vi "Graph Utilities Tree.vi"() -> ()   [LabVIEW 2016, in "graph_utilities.lvclass"]
uses:
  graph_utilities.lvclass
  graph_utilities.lvclass/graph_utilities.ctl
panel:
  out "XY Graph":cluster{"Intensity Data":dbl[], "Array":dbl[]}[](graph)
  out "Intensity Graph":dbl[][](graph)
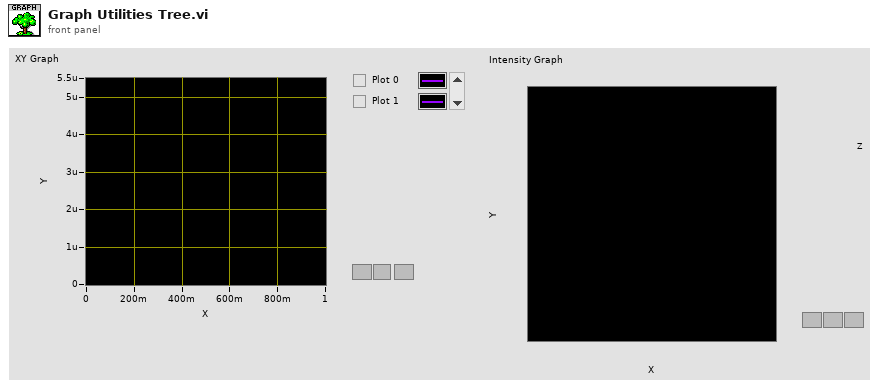
[diagram p1: front panel]
types:
  T1 = typedef "LVPointDoubleTypeDef.ctl" = cluster{"X":dbl, "Y":dbl}
  T2 = typedef "graph_utilities.lvclass/Scale Mapping  - Enum.ctl" = u16
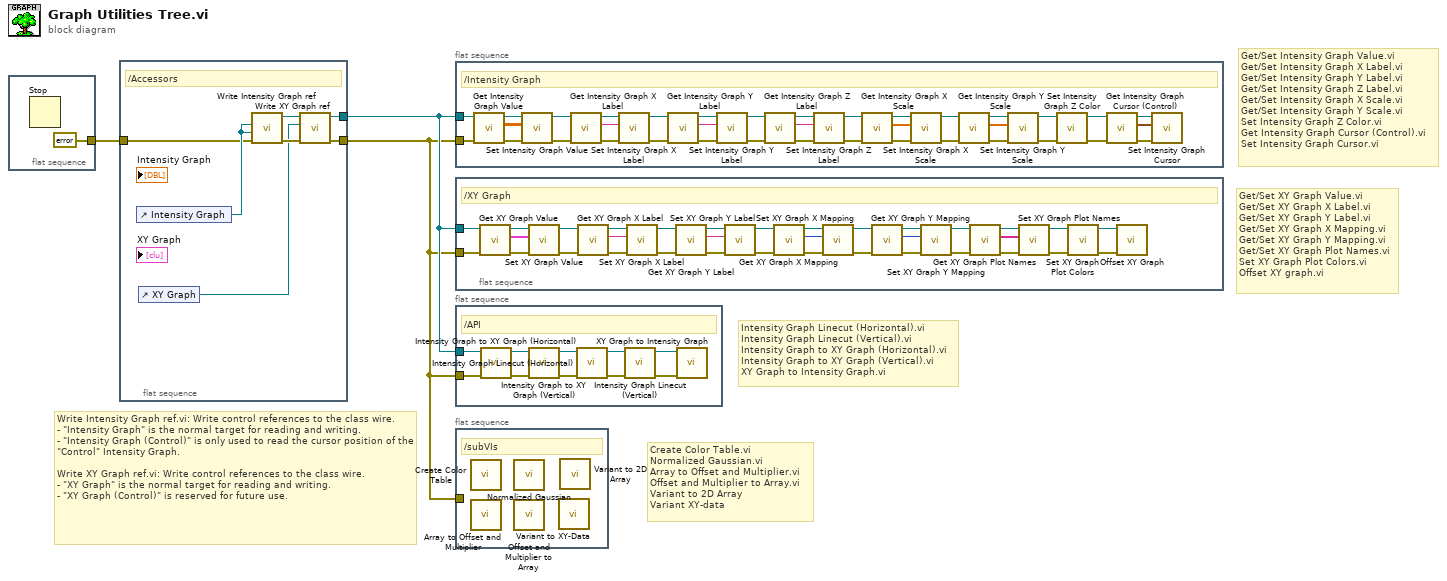
[diagram p0: block diagram]
diagram:
  # "Create Color Table.vi\nNormalized Gaussian.vi\nArray to Offset and Multiplier.vi\nOffset and Multiplier to Array.vi\nVariant to 2D Array\nVariant XY-data"
  # "Write Intensity Graph ref.vi: Write control references to the class wire.\n- \"Intensity Graph\" is the normal target for reading and writing.\n- \"Intensity Graph (Control)\" is only used to read the cursor position of the \"Control\" Intensity Graph.\n\nWrite XY Graph ref.vi: Write control references to the class wire.\n- \"XY Graph\" is the normal target for reading and writing.\n- \"XY Graph (Control)\" is reserved for future use."
  # "Get/Set Intensity Graph Value.vi\nGet/Set Intensity Graph X Label.vi\nGet/Set Intensity Graph Y Label.vi\nGet/Set Intensity Graph Z Label.vi\nGet/Set Intensity Graph X Scale.vi\nGet/Set Intensity Graph Y Scale.vi\nSet Intensity Graph Z Color.vi\nGet Intensity Graph Cursor (Control).vi\nSet Intensity Graph Cursor.vi"
  # "Get/Set XY Graph Value.vi\nGet/Set XY Graph X Label.vi\nGet/Set XY Graph Y Label.vi\nGet/Set XY Graph X Mapping.vi\nGet/Set XY Graph Y Mapping.vi\nGet/Set XY Graph Plot Names.vi\nSet XY Graph Plot Colors.vi\nOffset XY graph.vi"
  # "Intensity Graph Linecut (Horizontal).vi\nIntensity Graph Linecut (Vertical).vi\nIntensity Graph to XY Graph (Horizontal).vi\nIntensity Graph to XY Graph (Vertical).vi\nXY Graph to Intensity Graph.vi"
  n1 = flat-sequence {
    tunnel: [errorcluster {"status"=FALSE, "code"=0, "source"=""} ("error in (no error)")] -> w3
    frame #0 {
      n2 = Stop() -> ()  [unwired: 1 in]
    }
  }
  n3 = flat-sequence {
    tunnel: w3 -> [w7]
    tunnel: [w6] -> w2
    tunnel: [w5] -> w1
    frame #0 {
      # "/Accessors"
      n4 = control-ref of="Intensity Graph"() -> (w8:refnum<vi>)
      n5 = control-ref of="XY Graph"() -> (w9:refnum<vi>)
      n6 = call "Write Intensity Graph ref.vi"("error in (no error)"=w7, "Intensity Graph (Control)"=w8, "Intensity Graph"=w8) -> ("error out"=w10:errorcluster, "graph_utilities out"=w11:refnum<class "graph_utilities.lvclass">)  [unwired: 7 in]
      n7 = call "Write XY Graph ref.vi"("error in (no error)"=w10, "XY Graph"=w9, "graph_utilities in"=w11) -> ("error out"=w5:errorcluster, "graph_utilities out"=w6:refnum<class "graph_utilities.lvclass">)  [unwired: 7 in]
    }
  }
  n8 = flat-sequence {
    tunnel: w2 -> [w13]
    tunnel: w1 -> [w12]
    frame #0 {
      # "/Intensity Graph"
      n9 = call "Get Intensity Graph Value.vi"("error in (no error)"=w12, "graph_utilities in"=w13) -> ("error out"=w46:errorcluster, "Value"=w48:dbl[][], "graph_utilities out"=w47:refnum<class "graph_utilities.lvclass">)  [unwired: 7 in]
      n10 = call "Set Intensity Graph Value.vi"("error in (no error)"=w46, "Value"=w48, "graph_utilities in"=w47) -> ("error out"=w44:errorcluster, "graph_utilities out"=w45:refnum<class "graph_utilities.lvclass">)  [unwired: 7 in]
      n11 = call "Get Intensity Graph X Label.vi"("error in (no error)"=w44, "graph_utilities in"=w45) -> ("error out"=w42:errorcluster, "X Label"=w23:string, "graph_utilities out"=w43:refnum<class "graph_utilities.lvclass">)  [unwired: 7 in]
      n12 = call "Set Intensity Graph X Label.vi"("error in (no error)"=w42, "X Label"=w23, "graph_utilities in"=w43) -> ("error out"=w40:errorcluster, "graph_utilities out"=w41:refnum<class "graph_utilities.lvclass">)  [unwired: 7 in]
      n13 = call "Get Intensity Graph Y Label.vi"("error in (no error)"=w40, "graph_utilities in"=w41) -> ("error out"=w38:errorcluster, "Y Label"=w22:string, "graph_utilities out"=w39:refnum<class "graph_utilities.lvclass">)  [unwired: 7 in]
      n14 = call "Set Intensity Graph Y Label.vi"("error in (no error)"=w38, "Y Label"=w22, "graph_utilities in"=w39) -> ("error out"=w36:errorcluster, "graph_utilities out"=w37:refnum<class "graph_utilities.lvclass">)  [unwired: 7 in]
      n15 = call "Get Intensity Graph Z Label.vi"("error in (no error)"=w36, "graph_utilities in"=w37) -> ("error out"=w34:errorcluster, "Z Label"=w21:string, "graph_utilities out"=w35:refnum<class "graph_utilities.lvclass">)  [unwired: 7 in]
      n16 = call "Set Intensity Graph Z Label.vi"("error in (no error)"=w34, "Z Label"=w21, "graph_utilities in"=w35) -> ("error out"=w32:errorcluster, "graph_utilities out"=w33:refnum<class "graph_utilities.lvclass">)  [unwired: 7 in]
      n17 = call "Get Intensity Graph X Scale.vi"("error in (no error)"=w32, "graph_utilities in"=w33) -> ("error out"=w30:errorcluster, "X Scale"=w20:dbl[], "graph_utilities out"=w31:refnum<class "graph_utilities.lvclass">)  [unwired: 6 in, 1 out]
      n18 = call "Set Intensity Graph X Scale.vi"("error in (no error)"=w30, "X Scale"=w20, "graph_utilities in"=w31) -> ("error out"=w28:errorcluster, "graph_utilities out"=w29:refnum<class "graph_utilities.lvclass">)  [unwired: 7 in]
      n19 = call "Get Intensity Graph Y Scale.vi"("error in (no error)"=w28, "graph_utilities in"=w29) -> ("error out"=w26:errorcluster, "Y Scale"=w19:dbl[], "graph_utilities out"=w27:refnum<class "graph_utilities.lvclass">)  [unwired: 6 in, 1 out]
      n20 = call "Set Intensity Graph Y Scale.vi"("error in (no error)"=w26, "Y Scale"=w19, "graph_utilities in"=w27) -> ("error out"=w24:errorcluster, "graph_utilities out"=w25:refnum<class "graph_utilities.lvclass">)  [unwired: 7 in]
      n21 = call "Set Intensity Graph Z Color.vi"("error in (no error)"=w24, "graph_utilities in"=w25) -> ("error out"=w17:errorcluster, "graph_utilities out"=w16:refnum<class "graph_utilities.lvclass">)  [unwired: 8 in]
      n22 = call "Get Intensity Graph Cursor (Control).vi"("error in (no error)"=w17, "graph_utilities in"=w16) -> ("error out"=w15:errorcluster, "Cursor.Cursor Position"=w18:T1, "graph_utilities out"=w14:refnum<class "graph_utilities.lvclass">)  [unwired: 7 in]
      n23 = call "Set Intensity Graph Cursor.vi"("error in (no error)"=w15, "Cursor.Cursor Position"=w18, "graph_utilities in"=w14) -> ()  [unwired: 7 in, 2 out]
    }
  }
  n24 = flat-sequence {
    tunnel: w2 -> [w69]
    tunnel: w1 -> [w68]
    frame #0 {
      # "/XY Graph"
      n25 = call "Get XY Graph Value.vi"("error in (no error)"=w68, "graph_utilities in"=w69) -> ("error out"=w80:errorcluster, "Value"=w82:cluster{"X":dbl[], "Y":dbl[]}[], "graph_utilities out"=w81:refnum<class "graph_utilities.lvclass">)  [unwired: 7 in]
      n26 = call "Set XY Graph Value.vi"("error in (no error)"=w80, "Value"=w82, "graph_utilities in"=w81) -> ("error out"=w78:errorcluster, "graph_utilities out"=w79:refnum<class "graph_utilities.lvclass">)  [unwired: 7 in]
      n27 = call "Get XY Graph X Label.vi"("error in (no error)"=w78, "graph_utilities in"=w79) -> ("error out"=w76:errorcluster, "X Label"=w70:string, "graph_utilities out"=w77:refnum<class "graph_utilities.lvclass">)  [unwired: 7 in]
      n28 = call "Set XY Graph X Label.vi"("error in (no error)"=w76, "X Label"=w70, "graph_utilities in"=w77) -> ("error out"=w74:errorcluster, "graph_utilities out"=w75:refnum<class "graph_utilities.lvclass">)  [unwired: 7 in]
      n29 = call "Get XY Graph Y Label.vi"("error in (no error)"=w74, "graph_utilities in"=w75) -> ("error out"=w72:errorcluster, "Y Label"=w71:string, "graph_utilities out"=w73:refnum<class "graph_utilities.lvclass">)  [unwired: 7 in]
      n30 = call "Set XY Graph Y Label.vi"("error in (no error)"=w72, "Y Label"=w71, "graph_utilities in"=w73) -> ("error out"=w66:errorcluster, "graph_utilities out"=w67:refnum<class "graph_utilities.lvclass">)  [unwired: 7 in]
      n31 = call "Get XY Graph X Mapping.vi"("error in (no error)"=w66, "graph_utilities in"=w67) -> ("error out"=w64:errorcluster, "X Scale Mapping"=w51:T2, "graph_utilities out"=w65:refnum<class "graph_utilities.lvclass">)  [unwired: 7 in]
      n32 = call "Set XY Graph X Mapping.vi"("error in (no error)"=w64, "X Scale Mapping"=w51, "graph_utilities in"=w65) -> ("error out"=w62:errorcluster, "graph_utilities out"=w63:refnum<class "graph_utilities.lvclass">)  [unwired: 7 in]
      n33 = call "Get XY Graph Y Mapping.vi"("error in (no error)"=w62, "graph_utilities in"=w63) -> ("error out"=w60:errorcluster, "Y Scale Mapping"=w50:T2, "graph_utilities out"=w61:refnum<class "graph_utilities.lvclass">)  [unwired: 7 in]
      n34 = call "Set XY Graph Y Mapping.vi"("error in (no error)"=w60, "Y Scale Mapping"=w50, "graph_utilities in"=w61) -> ("error out"=w58:errorcluster, "graph_utilities out"=w59:refnum<class "graph_utilities.lvclass">)  [unwired: 7 in]
      n35 = call "Get XY Graph Plot Names.vi"("error in (no error)"=w58, "graph_utilities in"=w59) -> ("error out"=w56:errorcluster, "Plot Names []"=w49:string[], "graph_utilities out"=w57:refnum<class "graph_utilities.lvclass">)  [unwired: 7 in]
      n36 = call "Set XY Graph Plot Names.vi"("error in (no error)"=w56, "Plot Names []"=w49, "graph_utilities in"=w57) -> ("error out"=w54:errorcluster, "graph_utilities out"=w55:refnum<class "graph_utilities.lvclass">)  [unwired: 7 in]
      n37 = call "Set XY Graph Plot Colors.vi"("error in (no error)"=w54, "graph_utilities in"=w55) -> ("error out"=w52:errorcluster, "graph_utilities out"=w53:refnum<class "graph_utilities.lvclass">)  [unwired: 8 in]
      n38 = call "Offset XY Graph.vi"("error in (no error)"=w52, "graph_utilities in"=w53) -> ()  [unwired: 8 in, 2 out]
    }
  }
  n39 = flat-sequence {
    tunnel: w2 -> [w84]
    tunnel: w1 -> [w83]
    frame #0 {
      # "/API"
      n40 = call "Intensity Graph to XY Graph (Horizontal).vi"("error in (no error)"=w83, "graph_utilities in"=w84) -> ("error out"=w91:errorcluster, "graph_utilities out"=w92:refnum<class "graph_utilities.lvclass">)  [unwired: 8 in]
      n41 = call "Intensity Graph to XY Graph (Vertical).vi"("error in (no error)"=w91, "graph_utilities in"=w92) -> ("error out"=w89:errorcluster, "graph_utilities out"=w90:refnum<class "graph_utilities.lvclass">)  [unwired: 8 in]
      n42 = call "Intensity Graph Linecut (Horizontal).vi"("error in (no error)"=w89, "graph_utilities in"=w90) -> ("error out"=w87:errorcluster, "graph_utilities out"=w88:refnum<class "graph_utilities.lvclass">)  [unwired: 8 in]
      n43 = call "Intensity Graph Linecut (Vertical).vi"("error in (no error)"=w87, "graph_utilities in"=w88) -> ("error out"=w85:errorcluster, "graph_utilities out"=w86:refnum<class "graph_utilities.lvclass">)  [unwired: 8 in]
      n44 = call "XY Graph to Intensity Graph.vi"("error in (no error)"=w85, "graph_utilities in"=w86) -> ()  [unwired: 8 in, 2 out]
    }
  }
  n45 = flat-sequence {
    tunnel: w1 -> [_]
    frame #0 {
      # "/subVIs"
      n46 = call "Create Color Table.vi"() -> ()  [unwired: 2 in, 4 out]
      n47 = call "Array to Offset and Multiplier.vi"() -> ()  [unwired: 1 in, 1 out]
      n48 = call "Normalized Gaussian.vi"() -> ()  [unwired: 10 in, 2 out]
      n49 = call "Offset and Multiplier to Array.vi"() -> ()  [unwired: 2 in, 1 out]
      n50 = call "Variant to XY-Data.vi"() -> ()  [unwired: 2 in, 2 out]
      n51 = call "Variant to 2D Array.vi"() -> ()  [unwired: 2 in, 2 out]
    }
  }
